vi "Draw Filled Triangle.vi"(10 "Triangle":T1={"Vertex 1"={"Position"={"x"=0.0, "y"=0.0, "z"=0.0}, "UV"={"u"=0.0, "v"=0.0}, "Colour"=12517256}, "Vertex 2"={"Position"={"x"=0.0, "y"=0.0, "z"=0.0}, "UV"={"u"=0.0, "v"=0.0}, "Colour"=12517256}, "Vertex 3"={"Position"={"x"=0.0, "y"=0.0, "z"=0.0}, "UV"={"u"=0.0, "v"=0.0}, "Colour"=12517256}, "Colour"=0} {"Vertex 3"."UV"."v" min=0 max=1 step=0.1; "Vertex 3"."UV"."u" min=0 max=1 step=0.1; "Vertex 2"."UV"."v" min=0 max=1 step=0.1; "Vertex 2"."UV"."u" min=0 max=1 step=0.1; "Vertex 1"."UV"."v" min=0 max=1 step=0.1; "Vertex 1"."UV"."u" min=0 max=1 step=0.1}, 11 "Pixel Data in":u32[](array[numeric])) -> (3 "Pixel Data out":u32[](array[numeric]))   [LabVIEW 2020, in "Raster (FPGA).lvlib"]
uses:
  Raster (FPGA).lvlib
  Triangle.ctl
  Vertex.ctl
  Vector 3D.ctl
  UV.ctl
  Round Vertex.vi
  Calculate Line Reciprocal.vi
  Check Is Triangle Flat Bottomed.vi
panel:
  out "Top Vertex.Colour":u32(colorbox)
  # "(0,1)"
  # "(1,1)"
  # "(0,0)"
  # "(1,0)"
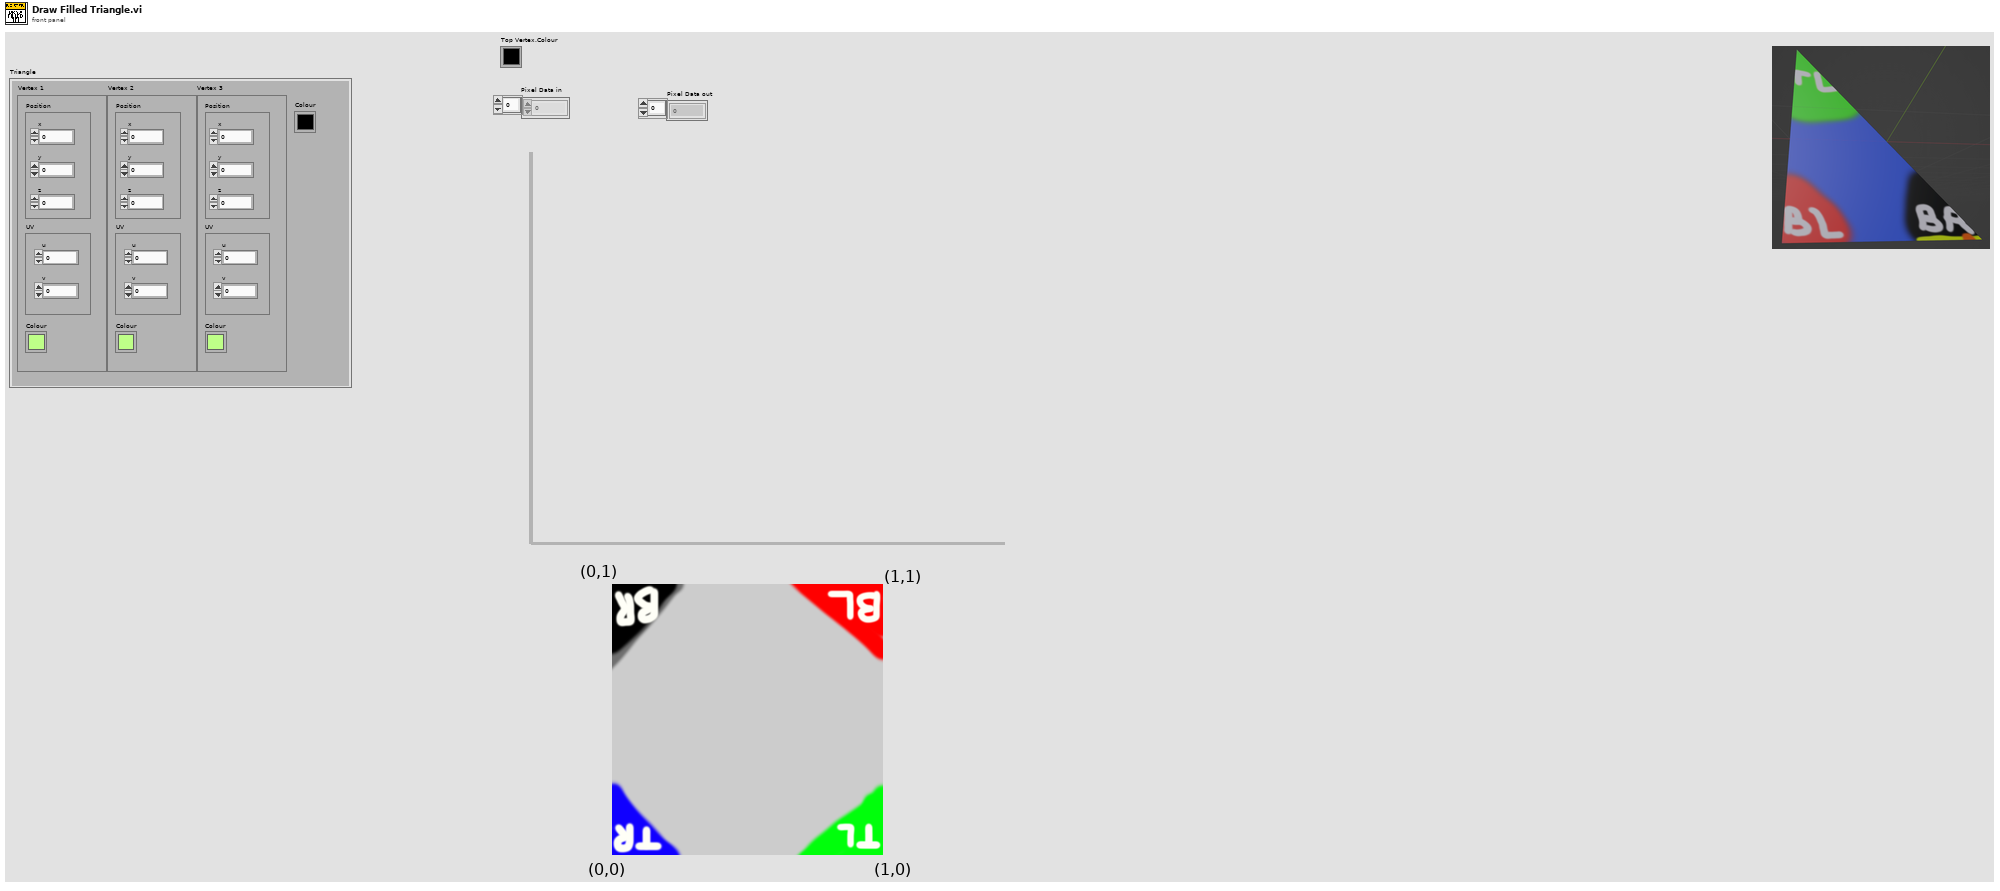
[diagram p1: front panel]
types:
  T1 = typedef "Raster (FPGA).lvlib/Triangle.ctl" = cluster{"Vertex 1":T2, "Vertex 2":T2, "Vertex 3":T2, "Colour":u32}
  T2 = typedef "Raster (FPGA).lvlib/Vertex.ctl" = cluster{"Position":T3, "UV":T4, "Colour":u32}
  T3 = typedef "Raster (FPGA).lvlib/Vector 3D.ctl" = cluster{"x":sgl, "y":sgl, "z":sgl}
  T4 = typedef "Raster (FPGA).lvlib/UV.ctl" = cluster{"u":sgl, "v":sgl}
  T5 = typedef "Raster (FPGA).lvlib/Triangle (Sorted).ctl" = cluster{"Top Vertex":T2, "Mid Vertex":T2, "Bottom Vertex":T2, "Colour":u32}
  T6 = typedef "Raster (FPGA).lvlib/Reciprocals.ctl" = cluster{"Bottom --> Top":sgl, "Bottom --> Middle":sgl, "Middle --> Top":sgl}
  T7 = typedef "Raster (FPGA).lvlib/Current Row.ctl" = cluster{"Start Column":sgl, "End Column":sgl}
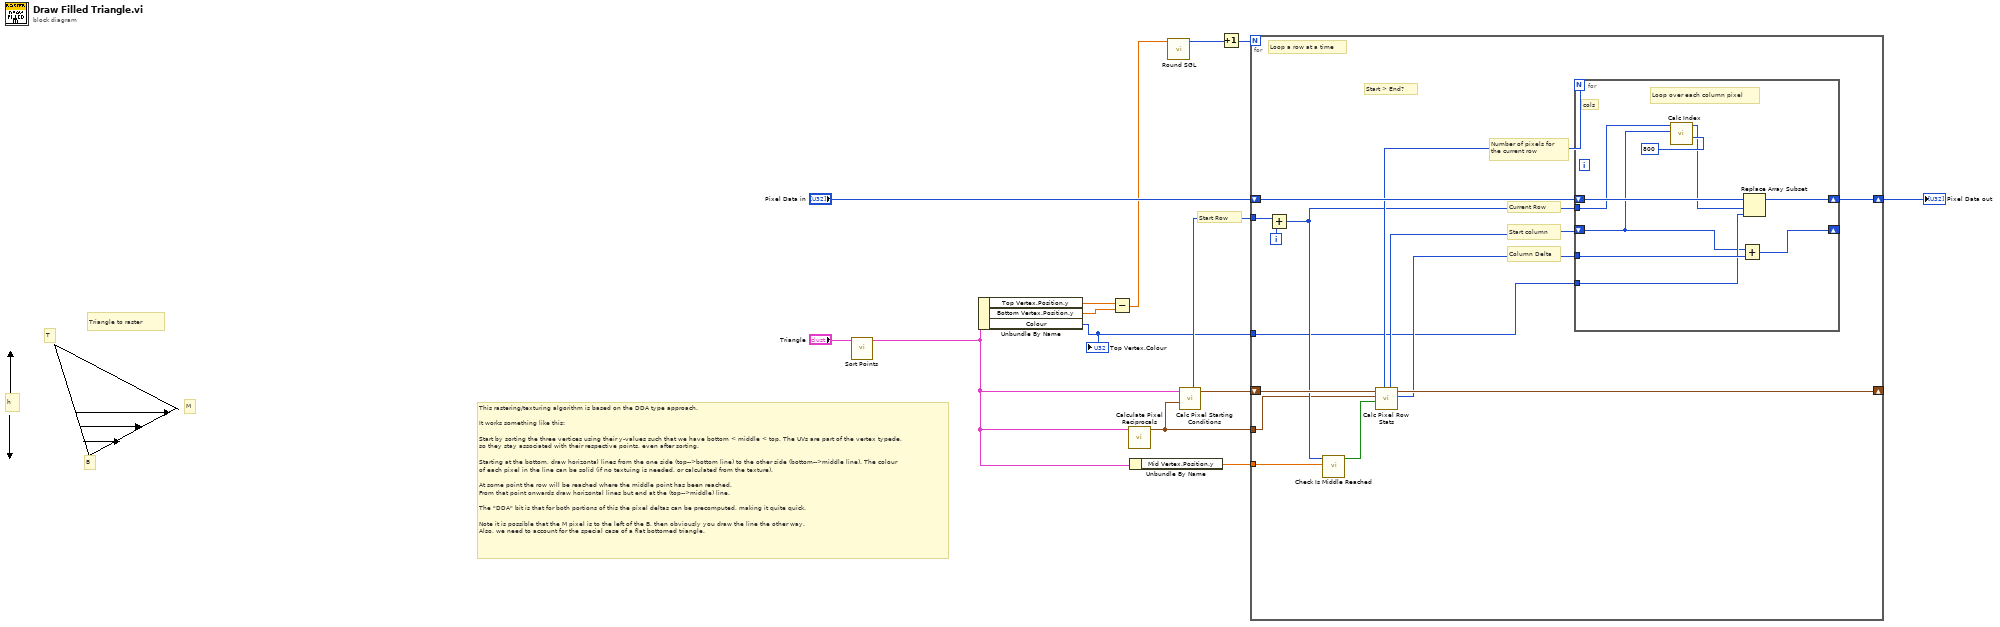
[diagram p0: block diagram]
diagram:
  # "h"
  # "Triangle to raster"
  # "M"
  # "T"
  # "B"
  # "This rastering/texturing algorithm is based on the DDA type approach.\n\nIt works something like this:\n\nStart by sorting the three vertices using their y-values such that we have bottom < middle < top. The UVs are part of the vertex typede, so they stay associated with their respective points, even after sorting.\n\nStarting at the bottom, draw horizontal lines from the one side (top-->bottom line) to the other side (bottom-->middle line). The colour of each pixel in the line can be solid (if no textuing is needed, or calculated from the texture).\n\nAt some point the row will be reached where the middle point has been reached.\nFrom that point onwards draw horizontal lines but end at the (top-->middle) line.\n\nThe \"DDA\" bit is that for both portions of this the pixel deltas can be precomputed, making it quite quick.\n\nNote it is possible that the M pixel is to the left of the B, then obviously you draw the line the other way.\nAlso, we need to account for the special case of a flat bottomed triangle."
  # "Start Row"
  n1 = call "Sort Points.vi"("Triangle"="Triangle") -> ("Sorted Triangle"=w4:T5)  [unwired: 10 in]
  n2 = Unbundle By Name(w4) -> ("Top Vertex.Position.y"=w8:sgl, "Bottom Vertex.Position.y"=w7:sgl, "Colour"=w3:u32)
  "Top Vertex.Colour" <- w3
  n3 = Subtract(x=w8, y=w7) -> (x-y=w2:sgl)
  n4 = call "Calculate Pixel Reciprocals.vi"("Sorted Triangle"=w4) -> ("Columns Pixels Per Row"=w12:T6)  [unwired: 10 in]
  n5 = Unbundle By Name(w4) -> ("Mid Vertex.Position.y"=w6:sgl)
  n6 = call "Round SGL.vi"("SGL"=w2) -> ("I32"=w1:i32)  [unwired: 10 in]
  n7 = call "Calc Pixel Starting Conditions.vi"("Reciprocals"=w12, "Sorted Vertices (V1 is top)"=w4) -> ("Start Row Columns"=w13:T7, "Start Row"=w14:i32)  [unwired: 8 in]
  n8 = Increment(x=w1) -> (x+1=w10:i32)
  n9 = for {
    N: w10 -> [_]
    shift-right: [w27] -> w9
    shift-left: "Pixel Data in" -> [w28]
    tunnel: w14 -> [w26]
    shift-right: [w22] -> _
    shift-left: w13 -> [w24]
    tunnel: w6 -> [w20]
    tunnel: w12 -> [w19]
    tunnel: w3 -> [w15]
    i -> [w25]
    # "Column Delta"
    # "Start > End?"
    # "Current Row"
    # "Start column"
    # "Loop a row at a time"
    # "Number of pixels for the current row"
    n10 = Add(x=w26, y=w25) -> (x+y=w21:i32)
    n11 = call "Check Is Middle Reached.vi"("Middle y"=w20, "Current Row"=w21) -> ("Reached Middle"=w18:bool)  [unwired: 9 in]
    n12 = call "Calc Pixel Row Stats.vi"("Reached Middle"=w18, "Reciprocals"=w19, "Current Row"=w24) -> ("Column Delta"=w17:i32, "Next Row"=w22:T7, "Start Col"=w16:i32, "Number Of Cols This Row"=w23:i32)  [unwired: 4 in, 1 out]
    n13 = for {
      N: w23 -> [_]
      shift-right: [w34] -> w27
      shift-left: w28 -> [w35]
      tunnel: w21 -> [w31]
      shift-right: [w37] -> _
      shift-left: w16 -> [w30]
      tunnel: w17 -> [w36]
      tunnel: w15 -> [w33]
      # "Loop over each column pixel"
      # "cols"
      n14 = call "Calc Index.vi"("Cols Per Row"=800, "Col"=w30, "Row"=w31) -> ("Index"=w29:i32)  [unwired: 8 in]
      n15 = Add(x=w30, y=w36) -> (x+y=w37:i32)
      n16 = Replace Array Subset(array=w35, new element=w33, index=w29) -> (w34:u32[])
    }
  }
  "Pixel Data out" <- w9
